vi "SPI Master with debug [FPGA].vi"() -> ()   [LabVIEW 2011]
uses:
  <vilib>/Platform/TimedLoop/XDataNode/timing_clust.ctl
  <vilib>/Platform/TimedLoop/XDataNode/nitl_modes.ctl
  <vilib>/Platform/TimedLoop/XDataNode/wakeup.ctl
  SPI Master State.ctl
  <vilib>/rvi/interface/RandomDataEmulation/nirviRandomDataFPGAFIFO.vi
  <vilib>/rvi/interface/RandomDataEmulation/niFpgaRandomDataHandleErrors.vi
  <vilib>/Platform/TimedLoop/XDataNode/XDataNode.xnode
  <vilib>/rvi/DataTransferAndStorage/Container/XNode/niFpgaContainer.xnode
  <vilib>/rvi/interface/RandomDataEmulation/nirviRandomDataFpgaReadWriteTemplate.vi
  <vilib>/Platform/TimedLoop/XDataNode/XDNodeRunTimeDep.lvlib
panel:
  in  "Data Length":u8
  in  "HCP-1":u8
  out "Data Out":u32
  in  "Data In":u32
  in  "TX":bool
  in  "CPOL":bool
  in  "CPHA":bool
  in  "RESET":bool
  out "_SS":bool
  out "SCLK":bool
  out "MOSI":bool
  in  "MISO":bool
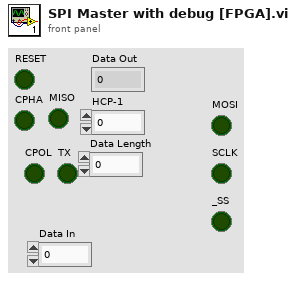
[diagram p1: front panel]
types:
  T1 = typedef "XDNodeRunTimeDep.lvlib/timing_clust.ctl" = cluster{"Expected End [f-1]":u64, "Actual End [f-1]":u64, "Finished Late? [f-1]":bool, "Expected End [i-1]":u64, "Actual End [i-1]":u64, "Finished Late? [i-1]":bool, "Expected Start [i]":u64, "Actual Start [i]":u64, "Expected Start [f]":u64, "Actual Start [f]":u64, "Source Name":string, "Structure Name":string, "Period":i64, "Deadline":i64, "Offset":i64, "Start":i64, "Priority":i32, "Timeout":i32, "Mode":T2, "Wakeup Reason":T3, "Error":errorcluster, "Source Type":string, "Secondary Source Type":string, "Global End Time":u64, "Global Start Time":u64, "Frame Duration":u64, "Iteration Duration":u64, "Assigned CPU":i32, "I/O Scan Engine Mode":u32}
  T2 = typedef "XDNodeRunTimeDep.lvlib/nitl_modes.ctl" = enum32{"No Change", "Process missed periods, maintain original phase", "Discard missed periods, maintain original phase", "Process missed periods, ignore original phase", "Discard missed periods, ignore original phase"}
  T3 = typedef "XDNodeRunTimeDep.lvlib/wakeup.ctl" = enum32{"Normal", "Aborted", "Asynchronous wakeup", "Timing source error", "Timed loop error", "Timeout"}
  T4 = typedef "SPI Master State.ctl" = enum8{"RESET", "Wait for TX", "Assert MOSI", "Toggle SCLK", "Latch MISO and Toggle SCLK", "Assert MOSI and Toggle SCLK"}
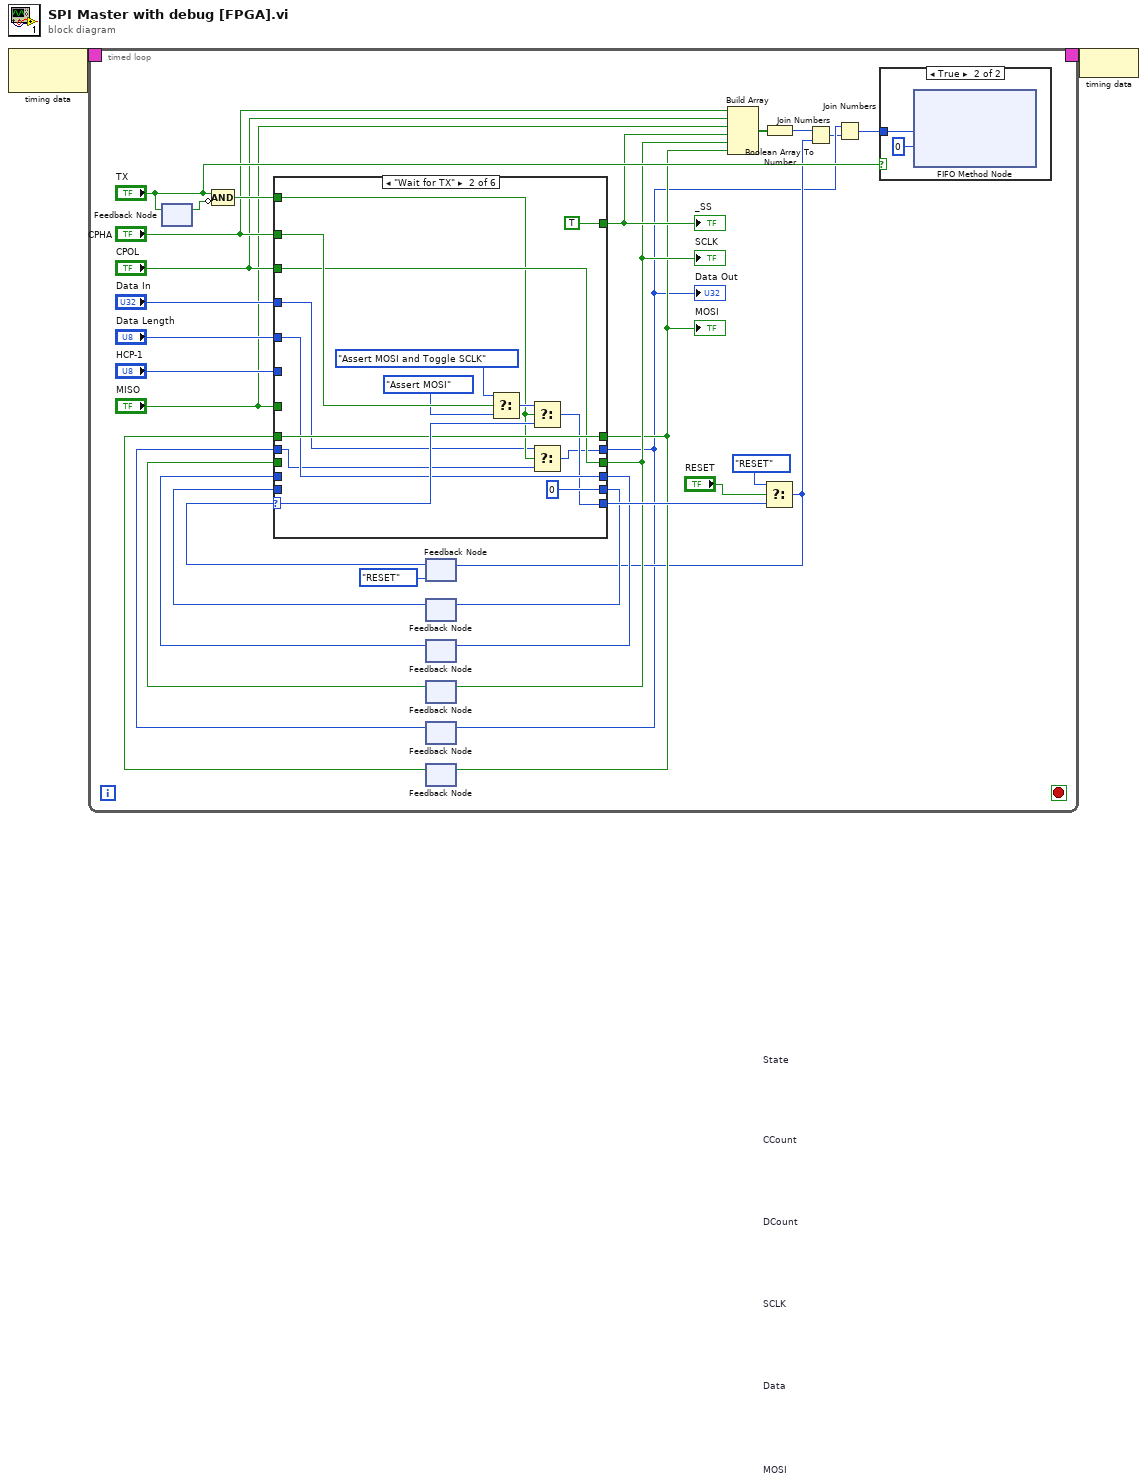
[diagram p0: block diagram]
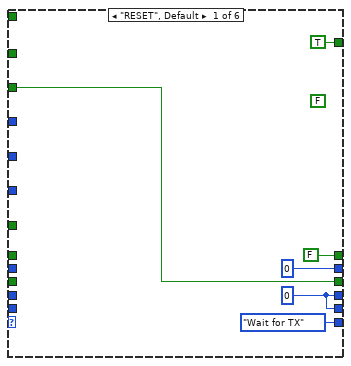
[diagram p3: hidden frame]
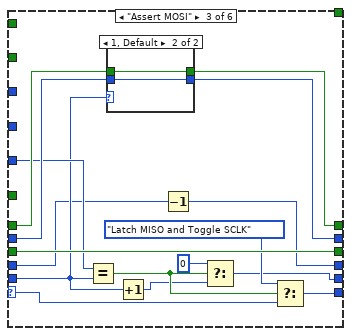
[diagram p4: hidden frame]
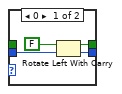
[diagram p5: hidden frame]
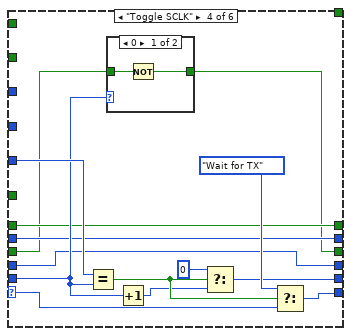
[diagram p6: hidden frame]
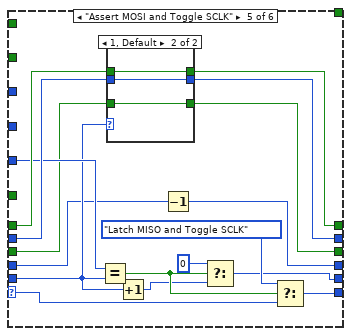
[diagram p8: hidden frame]
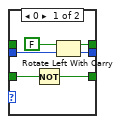
[diagram p9: hidden frame]
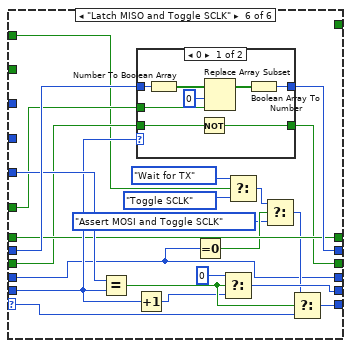
[diagram p10: hidden frame]
diagram:
  n1 = node-c288() -> (w2:T1)  [unwired: 1 in]
  n2 = timed-loop {
    timing: w2 -> [_]
    timing-out: [_] -> w1
    stop <- _ stop-if-true
    n3 = feedback #1() -> (w27:bool)  [unwired: 1 in]
    n4 = feedback-in #1("TX") -> ()
    n5 = Compound Arithmetic op=AND("TX", invert w27) -> (w19:bool)
    n6 = feedback #2 "State"(SPI_Master_State."RESET") -> (w31:T4)
    n7 = feedback #3 "CCount"() -> (w24:u8)  [unwired: 1 in]
    n8 = feedback #4 "DCount"() -> (w23:u8)  [unwired: 1 in]
    n9 = feedback #5 "SCLK"() -> (w22:bool)  [unwired: 1 in]
    n10 = feedback #6 "Data"() -> (w20:u32)  [unwired: 1 in]
    n11 = feedback #7 "MOSI"() -> (w18:bool)  [unwired: 1 in]
    n12 = case shown="\"Wait for TX\"" w31 {
      selector: w31 -> [_ w52 w64 w89 w105 w138]
      tunnel: [SPI_Master_State."Wait for TX" w45 w65 w90 w106 w139] -> w30
      tunnel: w19 -> [_ w44 _ _ _ _]
      tunnel: [w39 u8 0 w58 w83 w99 w133] -> w26
      tunnel: [w39 w47 w56 w82 w97 w121] -> w25
      tunnel: w24 -> [_ _ w61 w86 w102 w136]
      tunnel: w23 -> [_ _ w57 w82 w98 w121]
      tunnel: [TRUE ("MOSI") TRUE ("MOSI") _ _ _ _] -> w10
      tunnel: "CPHA" -> [_ w53 _ _ _ w127]
      tunnel: [w37 w46 w67 w78 w95 w129] -> w9
      tunnel: "CPOL" -> [w37 w46 _ _ _ _]
      tunnel: w22 -> [_ _ w67 w79 w96 w130]
      tunnel: "Data In" -> [_ w43 _ _ _ _]
      tunnel: [u32 0 ("Data In") w41 w70 w81 w110 w141] -> w4
      tunnel: w20 -> [_ w42 w71 w81 w111 w142]
      tunnel: "HCP-1" -> [_ _ w66 w91 w107 w140]
      tunnel: "MISO" -> [_ _ _ _ _ w131]
      tunnel: "Data Length" -> [_ w47 _ _ _ _]
      tunnel: [FALSE ("msb carry out") w48 w69 w80 w109 w132] -> w8
      tunnel: w18 -> [_ w48 w68 w80 w108 w132]
      frame "RESET", Default {
        (unwired) FALSE ("msb carry out")
        w39 = u8 0
      }
      frame "Wait for TX" {
        n13 = Select(t=SPI_Master_State."Assert MOSI and Toggle SCLK", s=w53, f=SPI_Master_State."Assert MOSI" ("t")) -> (s? t:f=w49:T4)
        n14 = Select(t=w49, s=w44, f=w52) -> (s? t:f=w45:T4)
        n15 = Select(t=w43, s=w44, f=w42) -> (s? t:f=w41:u32)
      }
      frame "Assert MOSI" {
        n16 = Equal?(x=w66, y=w61) -> (x = y?=w62:bool)
        n17 = case shown="1, Default" w61 {
          tunnel: w71 -> [w74 w76]
          tunnel: [w73 w76] -> w70
          tunnel: [w72 w77] -> w69
          tunnel: w68 -> [_ w77]
          frame 0 {
            n18 = Rotate Left With Carry(2:w74, 3:FALSE ("carry")) -> (0:w73:u32, 1:w72:bool)
          }
          frame 1, Default {
          }
        }
        n19 = Increment(x=w61) -> (x+1=w60:u8)
        n20 = Decrement(x=w57) -> (x-1=w56:u8)
        n21 = Select(t=u8 0, s=w62, f=w60) -> (s? t:f=w58:u8)
        n22 = Select(t=SPI_Master_State."Latch MISO and Toggle SCLK", s=w62, f=w64) -> (s? t:f=w65:T4)
      }
      frame "Toggle SCLK" {
        n23 = Equal?(x=w91, y=w86) -> (x = y?=w87:bool)
        n24 = case shown="0" w86 {
          tunnel: w79 -> [w93 w94]
          tunnel: [w92 w94] -> w78
          frame 0 {
            n25 = Not(x=w93) -> (.not. x?=w92:bool)
          }
          frame 1, Default {
          }
        }
        n26 = Increment(x=w86) -> (x+1=w85:u8)
        n27 = Select(t=u8 0, s=w87, f=w85) -> (s? t:f=w83:u8)
        n28 = Select(t=SPI_Master_State."Wait for TX", s=w87, f=w89) -> (s? t:f=w90:T4)
      }
      frame "Assert MOSI and Toggle SCLK" {
        n29 = Equal?(x=w107, y=w102) -> (x = y?=w103:bool)
        n30 = case shown="1, Default" w102 {
          tunnel: w111 -> [w116 w119]
          tunnel: [w115 w119] -> w110
          tunnel: [w114 w120] -> w109
          tunnel: w108 -> [_ w120]
          tunnel: w96 -> [w113 w118]
          tunnel: [w112 w118] -> w95
          frame 0 {
            n31 = Not(x=w113) -> (.not. x?=w112:bool)
            n32 = Rotate Left With Carry(2:w116, 3:FALSE ("carry")) -> (0:w115:u32, 1:w114:bool)
          }
          frame 1, Default {
          }
        }
        n33 = Increment(x=w102) -> (x+1=w101:u8)
        n34 = Decrement(x=w98) -> (x-1=w97:u8)
        n35 = Select(t=u8 0, s=w103, f=w101) -> (s? t:f=w99:u8)
        n36 = Select(t=SPI_Master_State."Latch MISO and Toggle SCLK", s=w103, f=w105) -> (s? t:f=w106:T4)
      }
      frame "Latch MISO and Toggle SCLK" {
        n37 = Equal?(x=w140, y=w136) -> (x = y?=w137:bool)
        n38 = Increment(x=w136) -> (x+1=w135:u8)
        n39 = case shown="0" w136 {
          tunnel: w142 -> [w150 w152]
          tunnel: [w145 w152] -> w141
          tunnel: w131 -> [w148 _]
          tunnel: w130 -> [w144 w151]
          tunnel: [w143 w151] -> w129
          frame 0 {
            n40 = Number To Boolean Array(number=w150) -> (Boolean array=w149:bool[])
            n41 = Not(x=w144) -> (.not. x?=w143:bool)
            n42 = Replace Array Subset(array=w149, new element=w148, index=0) -> (w146:bool[])
            n43 = Boolean Array To Number(Boolean array=w146) -> (number=w145:u32)
          }
          frame 1, Default {
          }
        }
        n44 = Equal To 0?(x=w121) -> (x = 0?=w128:bool)
        n45 = Select(t=u8 0, s=w137, f=w135) -> (s? t:f=w133:u8)
        n46 = Select(t=SPI_Master_State."Wait for TX", s=w127, f=SPI_Master_State."Toggle SCLK" ("t")) -> (s? t:f=w123:T4)
        n47 = Select(t=w123, s=w128, f=SPI_Master_State."Assert MOSI and Toggle SCLK" ("t")) -> (s? t:f=w125:T4)
        n48 = Select(t=w125, s=w137, f=w138) -> (s? t:f=w139:T4)
      }
    }
    "SCLK" <- w9
    "_SS" <- w10
    "MOSI" <- w8
    "Data Out" <- w4
    n49 = feedback-in #3(w26) -> ()
    n50 = feedback-in #4(w25) -> ()
    n51 = feedback-in #5(w9) -> ()
    n52 = feedback-in #6(w4) -> ()
    n53 = feedback-in #7(w8) -> ()
    n54 = Build Array("CPHA", "CPOL", "MISO", w10, w9, w8) -> (w7:bool[])
    n55 = Select(t=SPI_Master_State."RESET", s="RESET", f=w30) -> (s? t:f=w6:T4)
    n56 = feedback-in #2(w6) -> ()
    n57 = Boolean Array To Number(Boolean array=w7) -> (number=w5:u8)
    n58 = Join Numbers(hi=w5, lo=w6) -> ((hi.lo)=w3:u16)
    n59 = Join Numbers(hi=w4, lo=w3) -> ((hi.lo)=w14:u64)
    n60 = case shown="True" "TX" {
      tunnel: w14 -> [_ w33]
      frame False {
      }
      frame True {
        n61 = xnode ("FIFO Method Node")("Element"=w33, "Timeout"=0) -> ()  [unwired: 1 in, 2 out]
      }
    }
  }
  n62 = node-c288(w1) -> ()
